vi "TempConfigurationSubVI.vi"(8 "error in":errorcluster, 10 "Sim?":bool, 11 "physical channels":tag) -> (0 "error out":errorcluster, 3 "task out":refnum<k21>)   [LabVIEW 2017]
uses:
  <vilib>/DAQmx/configure/timing.llb/DAQmx Timing (Sample Clock).vi
  <vilib>/DAQmx/create/channels.llb/DAQmx Create Channel (AI-Voltage-Basic).vi
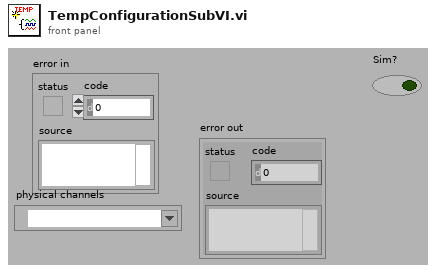
[diagram p1: front panel]
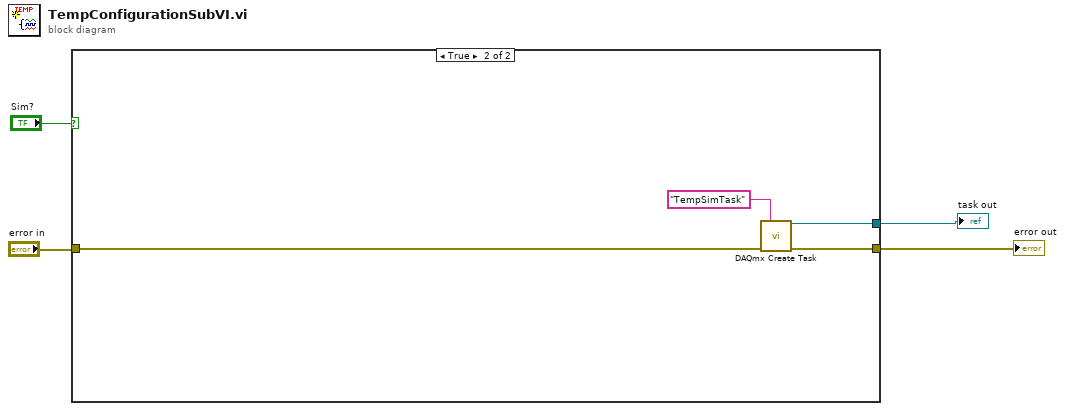
[diagram p0: block diagram]
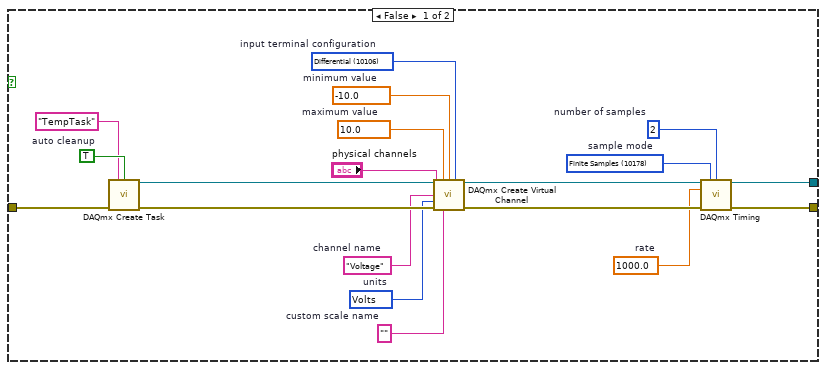
[diagram p2: hidden frame]
diagram:
  n1 = case shown="True" "Sim?" {
    tunnel: [w7 w27] -> w4
    tunnel: "error in" -> [w6 w26]
    tunnel: [w5 w24] -> w1
    frame False {
      w10 = 10178 items=["Finite Samples"=10178, "Continuous Samples"=10123, "Hardware Timed Single Point"=12522]  # sample mode
      w11 = 2  # number of samples
      w12 = 1000.0  # rate
      w14 = 10106 items=["default"=-1, "RSE"=10083, "NRSE"=10078, "Differential"=10106, "Pseudodifferential"=12529]  # input terminal configuration
      w15 = 10348 items=["Volts"=10348, "From Custom Scale"=10065]  # units
      w16 = "Voltage"  # channel name
      w18 = ""  # custom scale name
      w19 = -10.0  # minimum value
      w20 = 10.0  # maximum value
      w22 = TRUE  # auto cleanup
      n2 = call <vilib>:"DAQmx Create Task.vi"("new task name"="TempTask", "auto cleanup"=w22, "error in"=w6) -> ("task out"=w21:refnum<k21>, "error out"=w23:errorcluster)  [unwired: 11 in]
      n3 = call-poly <vilib>:"DAQmx Create Virtual Channel.vi"("task in"=w21, "maximum value"=w20, "minimum value"=w19, "input terminal configuration"=w14, "physical channels"="physical channels", "name to assign"=w16, "units"=w15, "error in"=w23, "custom scale name"=w18) -> ("task out"=w13:refnum<k21>, "error out"=w17:errorcluster)  [unwired: 5 in]
      n4 = call-poly <vilib>:"DAQmx Timing.vi"("task/channels in"=w13, "sample mode"=w10, "samples per channel"=w11, "rate"=w12, "error in"=w17) -> ("task out"=w5:refnum<k21>, "error out"=w7:errorcluster)  [unwired: 9 in]
    }
    frame True {
      n5 = call <vilib>:"DAQmx Create Task.vi"("new task name"="TempSimTask", "error in"=w26) -> ("task out"=w24:refnum<k21>, "error out"=w27:errorcluster)  [unwired: 12 in]
    }
  }
  "error out" <- w4
  "task out" <- w1
